vi "CAN_PID_Constants.vi"(11 "Control Mode":T1) -> (1 "D":dbl, 2 "I":dbl, 3 "P":dbl)   [LabVIEW 2009, in "OWNCAN.lvlib"]
uses:
  OWNCAN.lvlib
  CAN/SubVIs/CAN Jaguar Control Mode.ctl
  CAN.lvlib
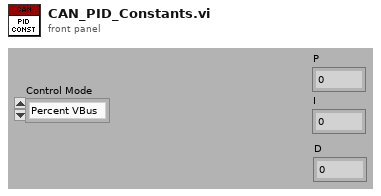
[diagram p1: front panel]
types:
  T1 = typedef "CAN.lvlib/CAN Jaguar Control Mode.ctl" = enum16{"Percent VBus", "Speed", "Position", "Current"}
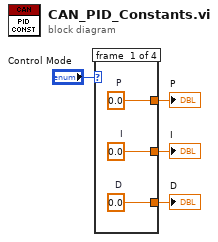
[diagram p0: block diagram]
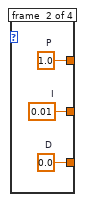
[diagram p2: hidden frame]
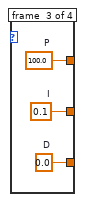
[diagram p3: hidden frame]
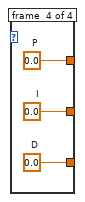
[diagram p4: hidden frame]
diagram:
  n1 = case shown="\"Current\"" "Control Mode" {
    tunnel: [w7 w10 w13 w16] -> w3
    tunnel: [w6 w9 w12 w15] -> w2
    tunnel: [w5 w8 w11 w14] -> w1
    frame #0 {
      w5 = 0.0  # D
      w6 = 0.0  # I
      w7 = 0.0  # P
    }
    frame #1 {
      w8 = 0.0  # D
      w9 = 0.01  # I
      w10 = 1.0  # P
    }
    frame #2 {
      w11 = 0.0  # D
      w12 = 0.1  # I
      w13 = 100.0  # P
    }
    frame #3 {
      w14 = 0.0  # D
      w15 = 0.0  # I
      w16 = 0.0  # P
    }
  }
  "P" <- w3
  "I" <- w2
  "D" <- w1
